vi "Add Library To Project.vi"(8 "error in":errorcluster, 9 "new library name":string, 10 "library path":path, 11 "project ref":refnum<vi>) -> (0 "error out":errorcluster, 3 "project ref out":refnum<vi>)   [LabVIEW 2021, in "MeasurementService Editor.lvlib"]
uses:
  MeasurementService Editor.lvlib
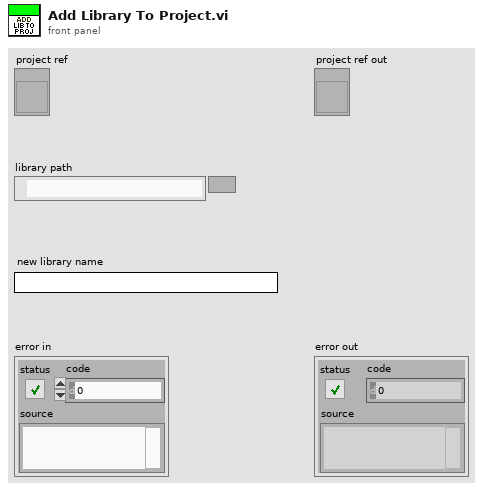
[diagram p1: front panel]
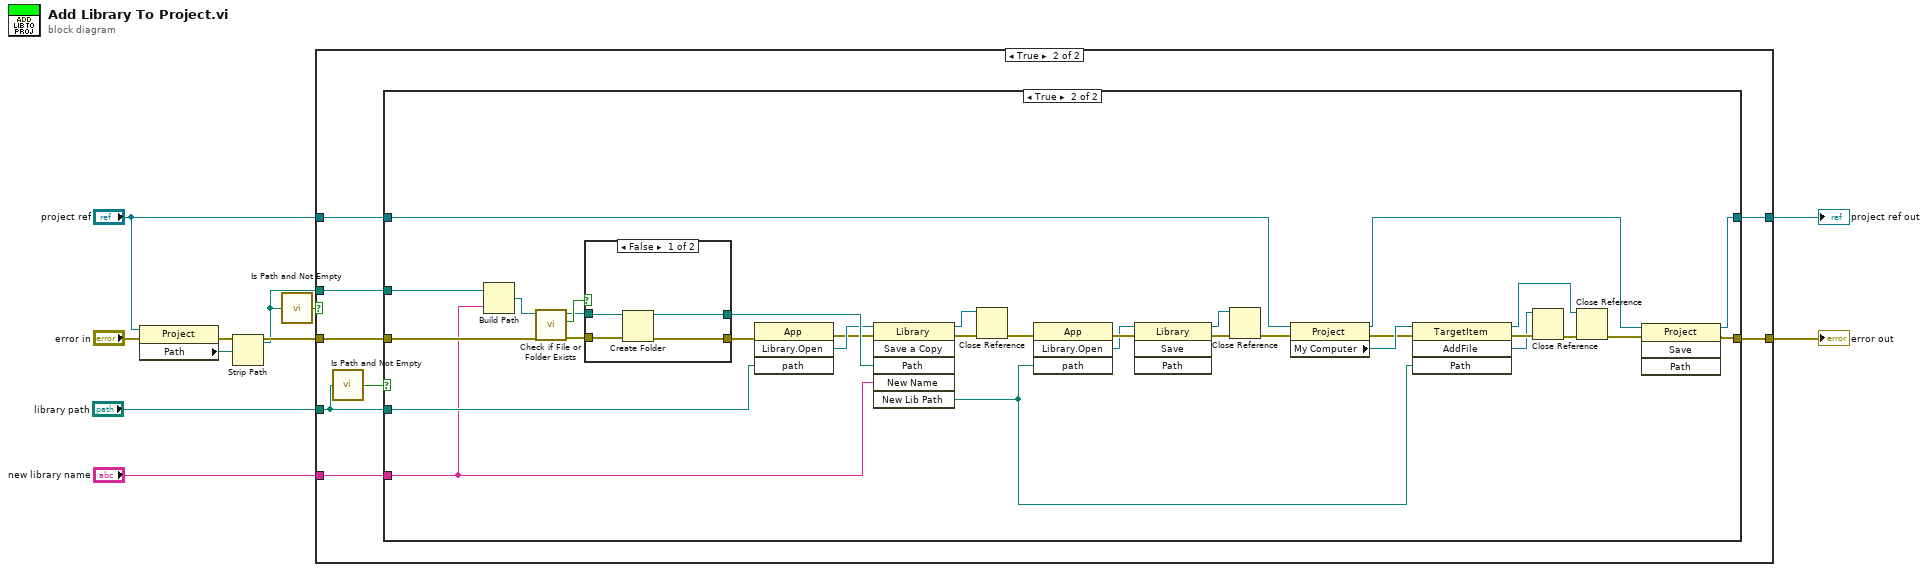
[diagram p0: block diagram]
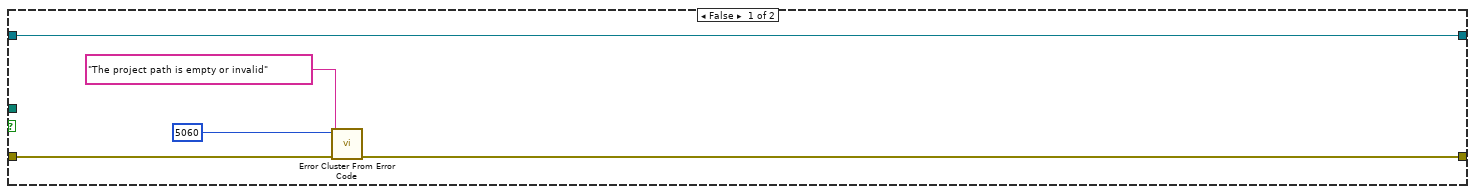
[diagram p2: hidden frame]
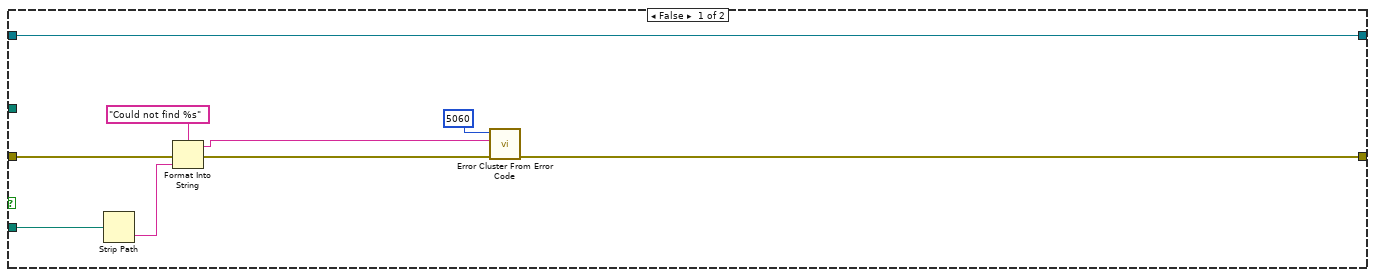
[diagram p3: hidden frame]
diagram:
  n1 = property class="Project"(reference="project ref", error in="error in") -> (error out=w7:errorcluster, "Path"=w4:path)  [unwired: 1 out]
  n2 = Strip Path(path=w4) -> (stripped path=w3:path)  [unwired: 1 out]
  n3 = call <vilib>:"Is Path and Not Empty.vi"("path"=w3) -> ("Is Path and Not Empty?"=w10:bool)  [unwired: 4 in]
  n4 = case shown="True" w10 {
    tunnel: w7 -> [w15 w23]
    tunnel: [w14 w22] -> w9
    tunnel: "library path" -> [_ w20]
    tunnel: "new library name" -> [_ w19]
    tunnel: w3 -> [_ w18]
    tunnel: "project ref" -> [w11 w17]
    tunnel: [w11 w16] -> w1
    frame False {
      n5 = call <vilib>:"Error Cluster From Error Code.vi"("error in (no error)"=w15, "error message (\"\")"="The project path is empty or invalid" ("error message (\"\")"), "error code (0)"=5060) -> ("error out"=w14:errorcluster)  [unwired: 6 in]
    }
    frame True {
      n6 = call <vilib>:"Is Path and Not Empty.vi"("path"=w20) -> ("Is Path and Not Empty?"=w21:bool)  [unwired: 4 in]
      n7 = case shown="True" w21 {
        tunnel: w23 -> [w31 w64]
        tunnel: [w30 w62] -> w22
        tunnel: w20 -> [w27 w63]
        tunnel: w19 -> [_ w53]
        tunnel: w18 -> [_ w61]
        tunnel: w17 -> [w24 w60]
        tunnel: [w24 w33] -> w16
        frame False {
          n8 = Strip Path(path=w27) -> (name=w28:string)  [unwired: 1 out]
          n9 = Format Into String(format string="Could not find %s", error in=w31, w28) -> (resulting string=w25:string, error out=w29:errorcluster)  [unwired: 1 in]
          n10 = call <vilib>:"Error Cluster From Error Code.vi"("error in (no error)"=w29, "error message (\"\")"=w25, "error code (0)"=5060) -> ("error out"=w30:errorcluster)  [unwired: 6 in]
        }
        frame True {
          n11 = Build Path(base path=w61, name or relative path=w53) -> (appended path=w59:path)
          n12 = call <vilib>:"Check if File or Folder Exists.vi"("error in (no error)"=w64, "path"=w59) -> ("error out"=w56:errorcluster, "file or folder exists?"=w58:bool, "dup path"=w57:path)  [unwired: 7 in]
          n13 = case shown="False" w58 {
            tunnel: w57 -> [w67 w70]
            tunnel: w56 -> [w68 w69]
            tunnel: [w66 w69] -> w55
            tunnel: [w65 w70] -> w54
            frame False {
              n14 = Create Folder(path (use dialog)=w67, error in=w68) -> (created path=w65:path, error out=w66:errorcluster)  [unwired: 1 in, 1 out]
            }
            frame True {
            }
          }
          n15 = invoke class="App" method="Library.Open"(error in=w55, "path"=w63) -> (error out=w40:errorcluster, "Open Library"=w52:refnum<vi>)  [unwired: 2 in, 2 out]
          n16 = invoke class="Library" method="Save a Copy"(reference=w52, error in=w40, "Path"=w54, "New Name"=w53) -> (reference out=w47:refnum<vi>, error out=w49:errorcluster, "New Lib Path"=w39:path)  [unwired: 2 in, 3 out]
          n17 = Close Reference(reference=w47, error in (no error)=w49) -> (error out=w48:errorcluster)
          n18 = invoke class="App" method="Library.Open"(error in=w48, "path"=w39) -> (error out=w35:errorcluster, "Open Library"=w34:refnum<vi>)  [unwired: 2 in, 2 out]
          n19 = invoke class="Library" method="Save"(reference=w34, error in=w35) -> (reference out=w45:refnum<vi>, error out=w46:errorcluster)  [unwired: 2 in, 2 out]
          n20 = Close Reference(reference=w45, error in (no error)=w46) -> (error out=w44:errorcluster)
          n21 = property class="Project"(reference=w60, error in=w44) -> (reference out=w41:refnum<vi>, error out=w50:errorcluster, "My Computer"=w51:refnum<vi>)
          n22 = invoke class="TargetItem" method="AddFile"(reference=w51, error in=w50, "Path"=w39) -> (reference out=w36:refnum<vi>, error out=w43:errorcluster, "AddFile"=w42:refnum<vi>)  [unwired: 1 in, 1 out]
          n23 = Close Reference(reference=w42, error in (no error)=w43) -> (error out=w38:errorcluster)
          n24 = Close Reference(reference=w36, error in (no error)=w38) -> (error out=w37:errorcluster)
          n25 = invoke class="Project" method="Save"(reference=w41, error in=w37) -> (reference out=w33:refnum<vi>, error out=w62:errorcluster)  [unwired: 2 in, 2 out]
        }
      }
    }
  }
  "error out" <- w9
  "project ref out" <- w1
